vi "fitROI_action.vi"(0 "HGF_ImaqFg in":refnum<class "HGF_ImaqFg.lvclass">, 1 "Region of Interest In":i32[](array[numeric]), 2 "Fit Mode":u32(ring) items=["Larger", "Smaller"], 5 "error in (no error)":errorcluster) -> (14 "HGF_ImaqFg out":refnum<class "HGF_ImaqFg.lvclass">, 15 "Region of Interest Out":i32[](array[numeric]), 19 "error out":errorcluster)   [LabVIEW 2014, in "HGF_IMAQ.lvlib" / "HGF_ImaqFg.lvclass"]
doc: "Evaluates the region of interest (ROI) you specify, and returns valid left, top, height, and width values."
uses:
  HGF_ImaqFg.lvclass
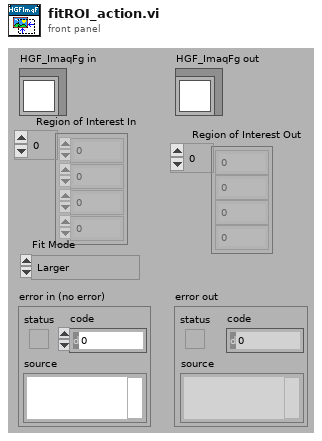
[diagram p1: front panel]
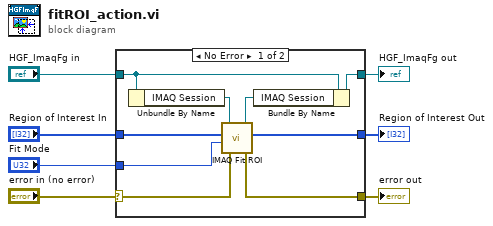
[diagram p0: block diagram]
diagram:
  n1 = case shown="No Error" "error in (no error)" {
    selector: "error in (no error)" -> [w8 w18]
    tunnel: [w16 w18] -> w7
    tunnel: "Region of Interest In" -> [w15 w17]
    tunnel: "Fit Mode" -> [w13 _]
    tunnel: [w12 w17] -> w4
    tunnel: "HGF_ImaqFg in" -> [w11 w19]
    tunnel: [w9 w19] -> w2
    frame No Error {
      n2 = Unbundle By Name(w11) -> ("IMAQ Session"=w14:refnum<k11>)
      n3 = call <vilib>:"IMAQ Fit ROI.vi"("error in (no error)"=w8, "Fit Mode"=w13, "Region of Interest In"=w15, "IMAQ Session In"=w14) -> ("error out"=w16:errorcluster, "Region of Interest Out"=w12:i32[], "IMAQ Session Out"=w10:refnum<k11>)  [unwired: 1 out]
      n4 = Bundle By Name(cluster=w11, "IMAQ Session"=w10) -> (w9:refnum<class "HGF_ImaqFg.lvclass">)
    }
    frame Error {
    }
  }
  "error out" <- w7
  "HGF_ImaqFg out" <- w2
  "Region of Interest Out" <- w4
